vi "Plugin.UDP.Get Connection IDs.vi"(11 "UDP Plugin in":refnum<class "UDP Plugin.lvclass">) -> (2 "connection IDs":refnum<k16>[](array[refnum]), 3 "UDP Plugin out":refnum<class "UDP Plugin.lvclass">)   [LabVIEW 2016, in "UDP Plugin.lvclass"]
uses:
  UDP Plugin.lvclass
  UDP Plugin.lvclass/UDP Plugin.ctl
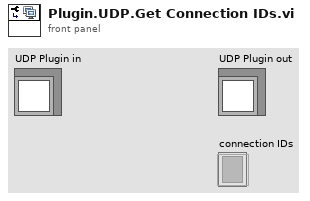
[diagram p1: front panel]
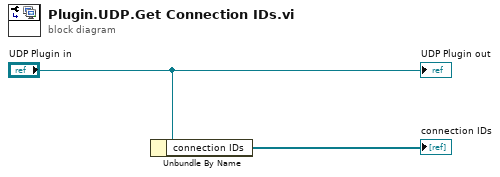
[diagram p0: block diagram]
diagram:
  n1 = Unbundle By Name("UDP Plugin in") -> ("connection IDs"=→"connection IDs":refnum<k16>[])
  "UDP Plugin out" <- "UDP Plugin in"
